vi "Axis Deadzone.vi"(1 "DeadZone Percent (Default 4)":dbl=4.0, 2 "Input":dbl) -> (0 "Output":dbl)   [LabVIEW 2014]
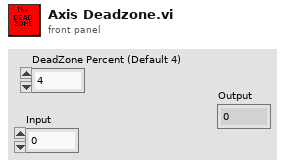
[diagram p1: front panel]
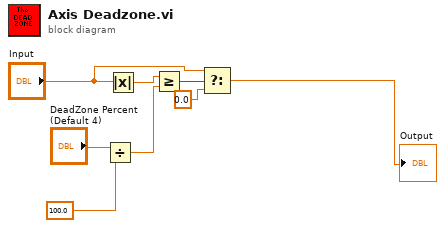
[diagram p0: block diagram]
diagram:
  n1 = Divide(x="DeadZone Percent (Default 4)", y=100.0) -> (x/y=w1:dbl)
  n2 = Absolute Value(x="Input") -> (abs(x)=w8:dbl)
  n3 = Greater Or Equal?(x=w8, y=w1) -> (x >= y?=w7:bool)
  n4 = Select(t="Input", s=w7, f=0.0) -> (s? t:f=→"Output":dbl)
